vi "Communication Manager.vi"(7 "Load?":bool, 8 "error in":errorcluster, 9 ">>ErrorQ":refnum<queue>, 11 ">>EventHandlers":refnum<user-event>) -> (0 "error out":errorcluster, 3 "Messaging Structures":T1)   [LabVIEW 2020, in "UserConsole.lvlib"]
doc: "Stores references to external communication structures for the module"
uses:
  UserConsole.lvlib
  Controls/Module Messaging Structures.ctl
  Support/Controls/Project Event Msg.ctl
  Support/Controls/Project Events.ctl
  Error Handler/Controls/Error QMsg.ctl
  Support/Controls/Project Modules.ctl
  Error Handler/ErrorHandler.lvlib
  Support/Support.lvlib
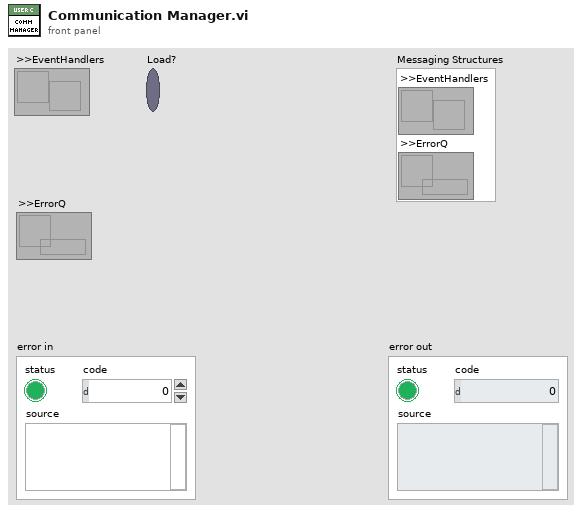
[diagram p1: front panel]
types:
  T1 = typedef "UserConsole.lvlib/Module Messaging Structures.ctl" = cluster{">>EventHandlers":refnum<user-event>, ">>ErrorQ":refnum<queue>}
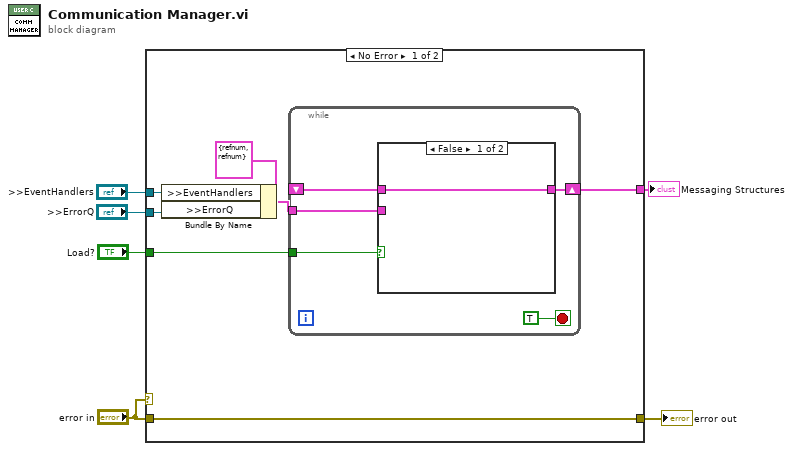
[diagram p0: block diagram]
diagram:
  n1 = case shown="No Error" "error in" {
    tunnel: "error in" -> [w12 w21]
    tunnel: [w12 w21] -> w5
    tunnel: [w9 _] -> w4
    tunnel: ">>ErrorQ" -> [w11 _]
    tunnel: ">>EventHandlers" -> [w10 _]
    tunnel: "Load?" -> [w7 _]
    frame No Error {
      n2 = Bundle By Name(cluster=T1 {">>EventHandlers"=refnum, ">>ErrorQ"=refnum} ("Messaging Structures"), ">>EventHandlers"=w10, ">>ErrorQ"=w11) -> (w8:T1)
      n3 = while {
        shift-right: [w17] -> w9
        shift-left: _ -> [w16]
        tunnel: w8 -> [w15]
        tunnel: w7 -> [w14]
        stop <- TRUE stop-if-true
        n4 = case shown="False" w14 {
          tunnel: [w19 w20] -> w17
          tunnel: w16 -> [w19 _]
          tunnel: w15 -> [_ w20]
          frame False {
          }
          frame True {
          }
        }
      }
    }
    frame Error {
    }
  }
  "error out" <- w5
  "Messaging Structures" <- w4
